vi "GetEV3_IP.vi"() -> (1 "Success?":bool, 3 "Info":T1)   [LabVIEW 2019]
panel:
  in  "Username":string="robot"
  in  "password":string="maker"
  in  "Cancel Button":bool
  in  "OK Button":bool
  in  "IP Address":string
  # "Setting up the EV3\n\n1. burn an SD Card from https://education.lego.com/en-us/support/mindstorms-ev3/python-for-ev3\n2. Start up your EV3 - and connect (https://www.ev3dev.org/docs/networking/)\n     a. connect up to the WiFi\n     b. use BT to share in internet connection (https://www.ev3dev.org/docs/tutorials/connecting-to-the-internet-via-bluetooth/)\n     c. use a hard wire connection (https://www.ev3dev.org/docs/tutorials/connecting-to-the-internet-via-usb/ )\n          Connect Cable to Mac/PC\n          On EV3 go to Wireless and Networks, All Network Connections, Wired, Connect\n          Wait a while for an IP Address - somethng like... - and Enter it below"
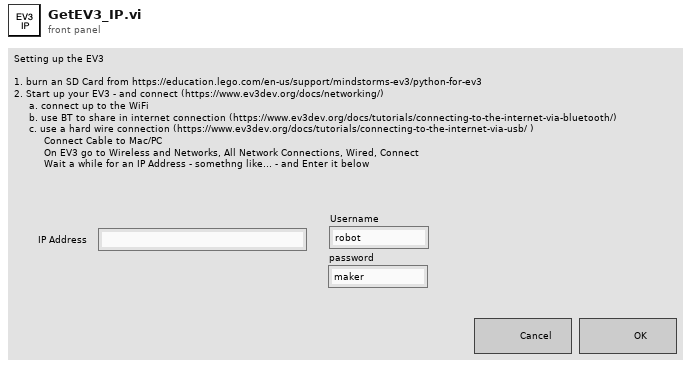
[diagram p1: front panel]
types:
  T1 = cluster{"IP Address":string, "Username":string, "password":string}
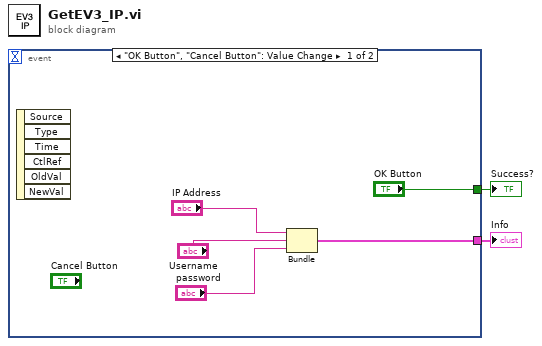
[diagram p0: block diagram]
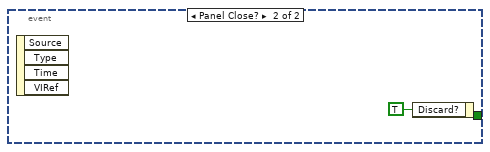
[diagram p2: hidden frame]
diagram:
  n1 = event shown="[0] \"OK Button\", \"Cancel Button\": Value Change" {
    selector: _ -> [_ _]
    dyn-events: _ -> [_ _]
    timeout: _ -> [_ _]
    tunnel: [w4 _] -> w2
    tunnel: ["OK Button" _] -> w1
    event "OK Button", "Cancel Button": Value Change {
      n2 = event-data() -> ()  [unwired: 1 in, 6 out]
      n3 = Bundle("IP Address"="IP Address", "Username"="Username", "password"="password") -> (w4:T1)  [unwired: 1 in]
    }
    event Panel Close? {
      n4 = event-data() -> ()  [unwired: 1 in, 4 out]
      n5 = event-data("Discard?"=TRUE) -> ()  [unwired: 1 in, 1 out]
    }
  }
  "Info" <- w2
  "Success?" <- w1
